vi "Test ArduinoMicro.vi"(5 "Enable":bool=TRUE, 8 "error in":errorcluster, 11 "VISA resource name":refnum<visa-resource-name>="COM16") -> (0 "error out":errorcluster)   [LabVIEW 2017]
uses:
  kissia_ArduinoMicro Module.ctl
panel:
  out "Status":bool
  out "write string":string
  in  "VALVES":T1
  out "read string":string
  out "Timeout":bool
  in  "stop":bool
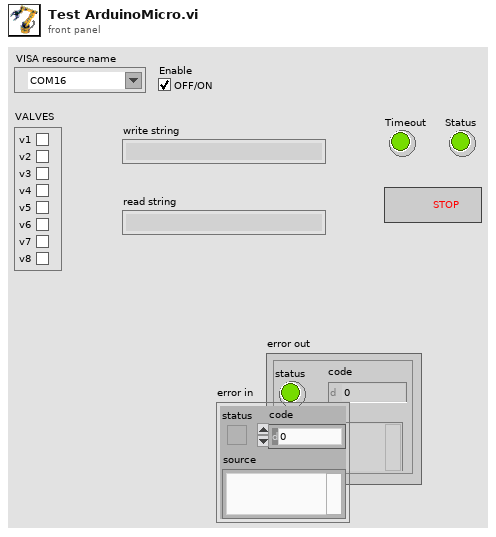
[diagram p1: front panel]
types:
  T1 = cluster{"v1":bool, "v2":bool, "v3":bool, "v4":bool, "v5":bool, "v6":bool, "v7":bool, "v8":bool}
  T2 = typedef "kissia_ArduinoMicro Module.ctl" = enum16{"Initialize", "Read Data", "Write Data", "Enable", "Disable", "Shutdown"}
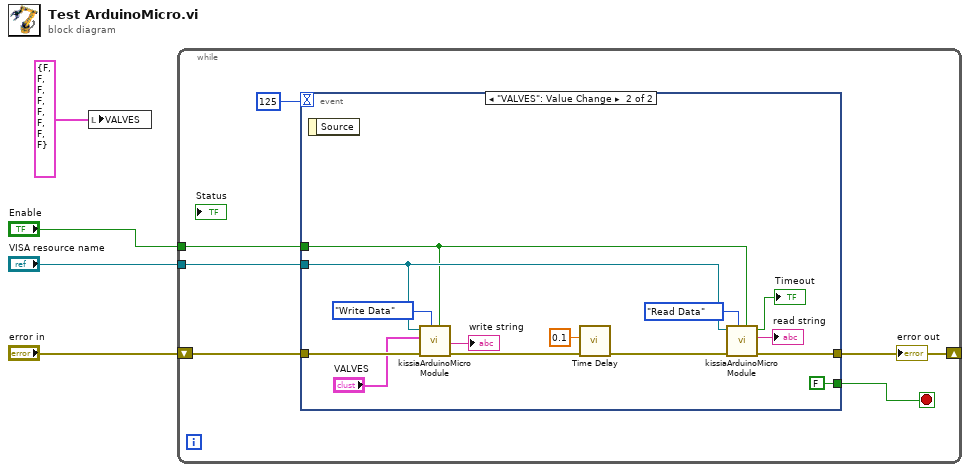
[diagram p0: block diagram]
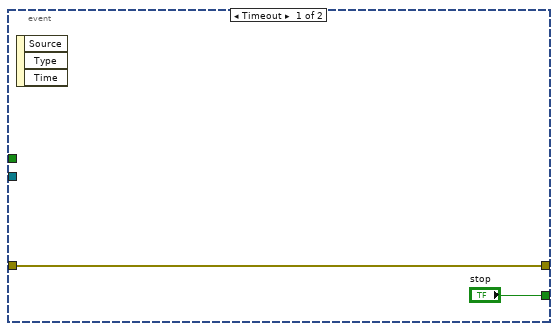
[diagram p2: hidden frame]
diagram:
  n1 = local write "VALVES"(T1 {"v1"=FALSE, "v2"=FALSE, "v3"=FALSE, "v4"=FALSE, "v5"=FALSE, "v6"=FALSE, "v7"=FALSE, "v8"=FALSE} ("VALVES")) -> ()
  n2 = while {
    shift-right: [w8] -> _
    shift-left: "error in" -> [w7]
    tunnel: "VISA resource name" -> [w9]
    tunnel: "Enable" -> [w10]
    stop <- w6 stop-if-true
    n3 = event shown="[1] \"VALVES\": Value Change" {
      selector: _ -> [_ _]
      dyn-events: _ -> [_ _]
      timeout: u32 125 ("milliseconds to wait") -> [_ _]
      tunnel: w10 -> [_ w17]
      tunnel: w9 -> [_ w18]
      tunnel: [w12 w16] -> w8
      tunnel: w7 -> [w12 w15]
      tunnel: ["stop" FALSE ("stop")] -> w6
      event Timeout {
        n4 = event-data() -> ()  [unwired: 1 in, 3 out]
      }
      event "VALVES": Value Change {
        n5 = event-data() -> ()  [unwired: 1 in, 1 out]
        n6 = call "kissiaArduinoMicro Module.vi"("Enable"=w17, "Command"=kissia_ArduinoMicro_Module."Write Data", "error in (no error)"=w15, "VALVES"="VALVES", "VISA resource name"=w18) -> ("error out"=w25:errorcluster, "write string"=→"write string":string)  [unwired: 3 in, 2 out]
        n7 = call "Time Delay"("error in (no error)"=w25, "Delay Time (s)"=0.1) -> ("error out"=w26:errorcluster)  [unwired: 9 in]
        n8 = call "kissiaArduinoMicro Module.vi"("Enable"=w17, "Command"=kissia_ArduinoMicro_Module."Read Data", "error in (no error)"=w26, "VISA resource name"=w18) -> ("error out"=w16:errorcluster, "read string"=→"read string":string, "TimeOut"=→"Timeout":bool)  [unwired: 4 in, 1 out]
      }
    }
    "error out" <- w8
  }
